vi "Configure -- subVI.vi"(8 "error in (no error)":errorcluster, 11 "VISA Refnum in":refnum<visa-resource-name>) -> (0 "error out":errorcluster)   [LabVIEW 2020, in "Lock-in amplifier.lvlib"]
uses:
  Lock-in amplifier.lvlib
  <instrlib>/Stanford Research 830/Stanford Research 830.lvlib
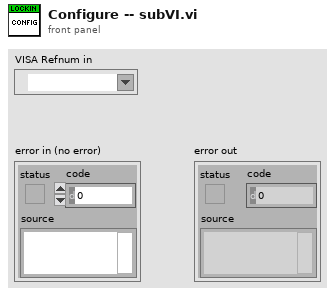
[diagram p1: front panel]
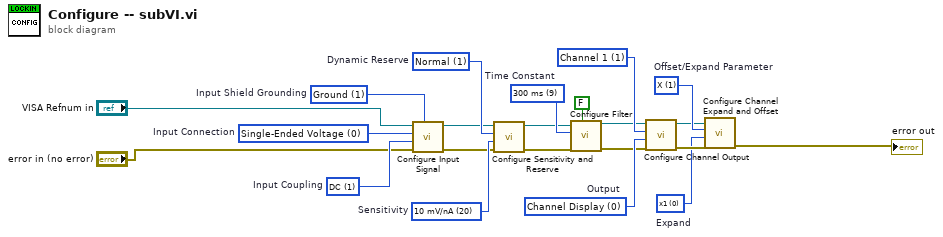
[diagram p0: block diagram]
diagram:
  w10 = i16 1 items=["Auto Reserve"=-1, "High Reserve"=0, "Normal"=1, "Low Noise"=2]  # Dynamic Reserve
  w11 = i16 20 items=["Auto Gain"=-1, "2 nV/fA"=0, "5 nV/fA"=1, "10 nV/fA"=2, "20 nV/fA"=3, "50 nV/fA"=4, "100 nV/fA"=5, "200 nV/fA"=6, "500 nV/fA"=7, "1 uV/pA"=8, "2 uV/pA"=9, "5 uV/pA"=10, "10 uV/pA"=11, "20 uV/pA"=12, "50 uV/pA"=13, "100 uV/pA"=14, "200 uV/pA"=15, "500 uV/pA"=16, "1 mV/nA"=17, "2 mV/nA"=18, "5 mV/nA"=19, "10 mV/nA"=20, "20 mV/nA"=21, "50 mV/nA"=22, "100 mV/nA"=23, "200 mV/nA"=24, "500 mV/mA"=25, "1 V/uA"=26]  # Sensitivity
  w12 = u16 9 items=["10 us", "30 us", "100 us", "300 us", "1 ms", "3 ms", "10 ms", "30 ms", "100 ms", "300 ms", "1 s", "3 s", "10 s", "30 s", "100 s", "300 s", "1 ks", "3 ks", "10 ks", "30 ks"]  # Time Constant
  w22 = u16 1 items=["X"=1, "Y"=2, "R"=3]  # Offset/Expand Parameter
  w19 = u16 0 items=["x1", "x10", "x100"]  # Expand
  w18 = u16 0 items=["Channel Display", "X or Y"]  # Output
  w17 = u16 1 items=["Channel 1"=1, "Channel 2"=2] ("Channel (1: Channel 1)")
  w15 = u16 1 items=["AC", "DC"]  # Input Coupling
  w14 = u16 0 items=["Single-Ended Voltage", "Differential Voltage", "1 MOhm Current Gain", "100 MOhm Current Gain"]  # Input Connection
  w13 = u16 1 items=["Float", "Ground"]  # Input Shield Grounding
  n1 = call <instrlib>:"Configure Input Signal.vi"("Input Shield Grounding (0: Float)"=w13, "error in (no error)"="error in (no error)", "Input Coupling (0: AC)"=w15, "Input Connection (0: Single-Ended Voltage)"=w14, "VISA resource name"="VISA Refnum in") -> ("error out"=w7:errorcluster, "VISA resource name out"=w6:refnum<visa-resource-name>)  [unwired: 5 in]
  n2 = call <instrlib>:"Configure Sensitivity and Reserve.vi"("error in (no error)"=w7, "Sensitivity (-1: Auto gain)"=w11, "Dynamic Reserve (-1: Auto Reserve)"=w10, "VISA resource name"=w6) -> ("error out"=w5:errorcluster, "VISA resource name out"=w4:refnum<visa-resource-name>)  [unwired: 6 in]
  n3 = call <instrlib>:"Configure Filter.vi"("Enable Sync Filter (F: Disable)"=FALSE, "error in (no error)"=w5, "Time Constant (8: 100ms)"=w12, "VISA resource name"=w4) -> ("error out"=w3:errorcluster, "VISA resource name out"=w2:refnum<visa-resource-name>)  [unwired: 6 in]
  n4 = call <instrlib>:"Configure Channel Output.vi"("error in (no error)"=w3, "Output (0: Channel Display)"=w18, "Channel (1: Channel 1)"=w17, "VISA resource name"=w2) -> ("error out"=w21:errorcluster, "VISA resource name out"=w20:refnum<visa-resource-name>)  [unwired: 6 in]
  n5 = call <instrlib>:"Configure Channel Expand and Offset.vi"("error in (no error)"=w21, "Expand (0: x1)"=w19, "Offset/Expand Parameter (1: X)"=w22, "VISA resource name"=w20) -> ("error out"=→"error out":errorcluster)  [unwired: 6 in, 1 out]
